vi "亂數產生器.vi"(1 "Min":dbl, 2 "Max":dbl) -> (0 "Random":dbl)   [LabVIEW 2014]
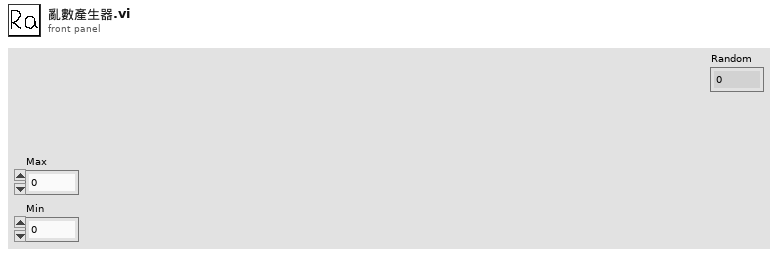
[diagram p1: front panel]
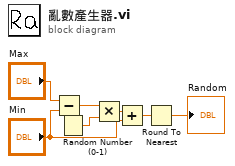
[diagram p0: block diagram]
diagram:
  n1 = Subtract(x="Max", y="Min") -> (x-y=w6:dbl)
  n2 = Random Number (0-1)() -> (number: 0 to 1=w5:dbl)
  n3 = Multiply(x=w6, y=w5) -> (x*y=w4:dbl)
  n4 = Add(x=w4, y="Min") -> (x+y=w2:dbl)
  n5 = Round To Nearest(number=w2) -> (nearest integer value=→"Random":dbl)
